vi "check folders.vi"(8 "error in (no error)":errorcluster, 11 "small stitch path":path) -> (0 "error out":errorcluster)   [LabVIEW 2012]
panel:
  out "max 2nd dimension":i32
  out "2nd dimensions":i32[](array[numeric])
  out "1st dimension":i32
  out "2nd coordinate array":string[][](array[string])
  out "1st coordinate array":string[](array[string])
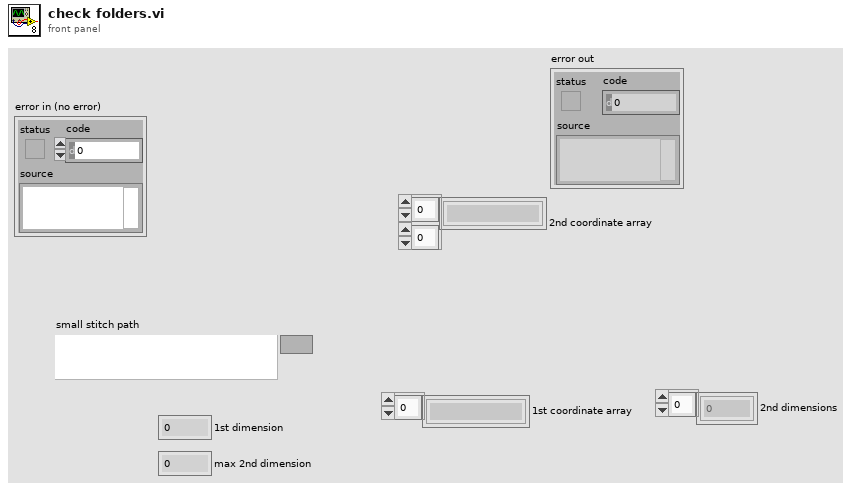
[diagram p1: front panel]
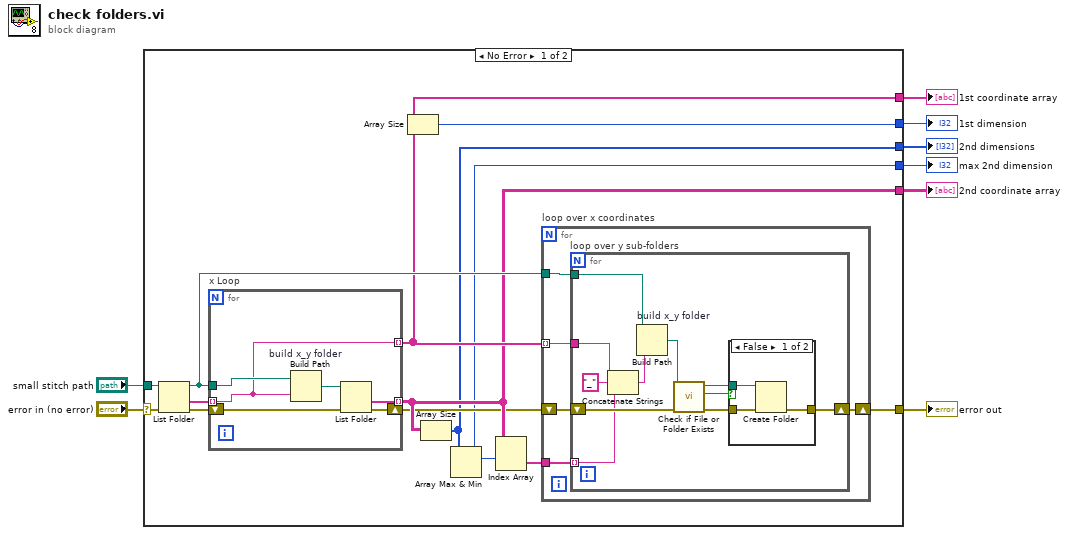
[diagram p0: block diagram]
diagram:
  n1 = case shown="No Error" "error in (no error)" {
    selector: "error in (no error)" -> [w21 w49]
    tunnel: "small stitch path" -> [w22 _]
    tunnel: [w17 w49] -> w6
    tunnel: [w16 _] -> w5
    tunnel: [w15 _] -> w4
    tunnel: [w14 _] -> w3
    tunnel: [w10 _] -> w2
    tunnel: [w9 _] -> w1
    frame No Error {
      n2 = List Folder(path=w22, error in=w21) -> (path out=w18:path, folder names=w20:string[], error out=w19:errorcluster)  [unwired: 2 in, 1 out]
      n3 = for "x Loop" {
        shift-right: [w45] -> w11
        shift-left: w19 -> [w47]
        tunnel: w20 -> [w44] mode=indexing
        tunnel: w18 -> [w48]
        tunnel: [w44] -> w15 mode=indexing
        tunnel: [w43] -> w14 mode=indexing
        n4 = Build Path "build x_y folder"(base path=w48, name or relative path=w44) -> (appended path=w46:path)
        n5 = List Folder(path=w46, error in=w47) -> (folder names=w43:string[], error out=w45:errorcluster)  [unwired: 2 in, 2 out]
      }
      n6 = Array Size(array=w15) -> (size(s)=w16:i32)
      n7 = Array Size(array=w14) -> (size(s)=w10:i32[])
      n8 = Array Max & Min(array=w10) -> (max value=w9:i32, max index (indices)=w13:i32)  [unwired: 2 out]
      n9 = Index Array(array=w14, index (row)=w13) -> (element=w12:string[])  [unwired: 1 in]
      n10 = for "loop over x coordinates" {
        tunnel: w15 -> [w25] mode=indexing
        shift-right: [w23] -> w17
        shift-left: w11 -> [w27]
        tunnel: w18 -> [w26]
        tunnel: w12 -> [w24]
        n11 = for "loop over y sub-folders" {
          tunnel: w26 -> [w34]
          tunnel: w25 -> [w32]
          tunnel: w24 -> [w30] mode=indexing
          shift-right: [w28] -> w23
          shift-left: w27 -> [w35]
          n12 = Concatenate Strings(w32, "_" ("string"), w30) -> (w31:string)
          n13 = Build Path "build x_y folder"(base path=w34, name or relative path=w31) -> (appended path=w29:path)
          n14 = call <vilib>:"Check if File or Folder Exists.vi"("error in (no error)"=w35, "path"=w29) -> ("error out"=w37:errorcluster, "file or folder exists?"=w36:bool, "dup path"=w38:path)  [unwired: 7 in]
          n15 = case shown="False" w36 {
            tunnel: w37 -> [w41 w42]
            tunnel: [w40 w42] -> w28
            tunnel: w38 -> [w39 _]
            frame False {
              n16 = Create Folder(path (use dialog)=w39, error in=w41) -> (error out=w40:errorcluster)  [unwired: 1 in, 2 out]
            }
            frame True {
            }
          }
        }
      }
    }
    frame Error {
    }
  }
  "error out" <- w6
  "1st dimension" <- w5
  "1st coordinate array" <- w4
  "2nd coordinate array" <- w3
  "2nd dimensions" <- w2
  "max 2nd dimension" <- w1
